vi "H.Signal.vi"() -> (2 "element":bool, 4 "Slide servo home RS":bool, 6 "HI Bit Auto":bool, 8 "Error M Auto":string, 10 "Error Message":string, 15 "Bool_H Sig":bool)   [LabVIEW 2015]
uses:
  Galobal variable_TI.vi
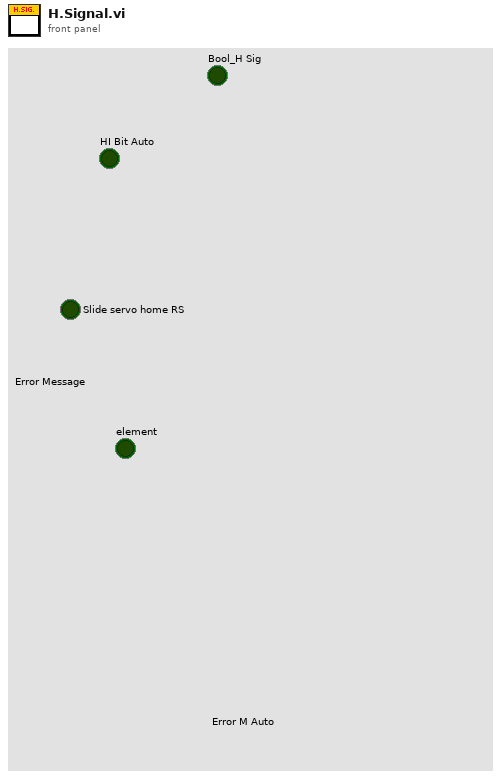
[diagram p1: front panel]
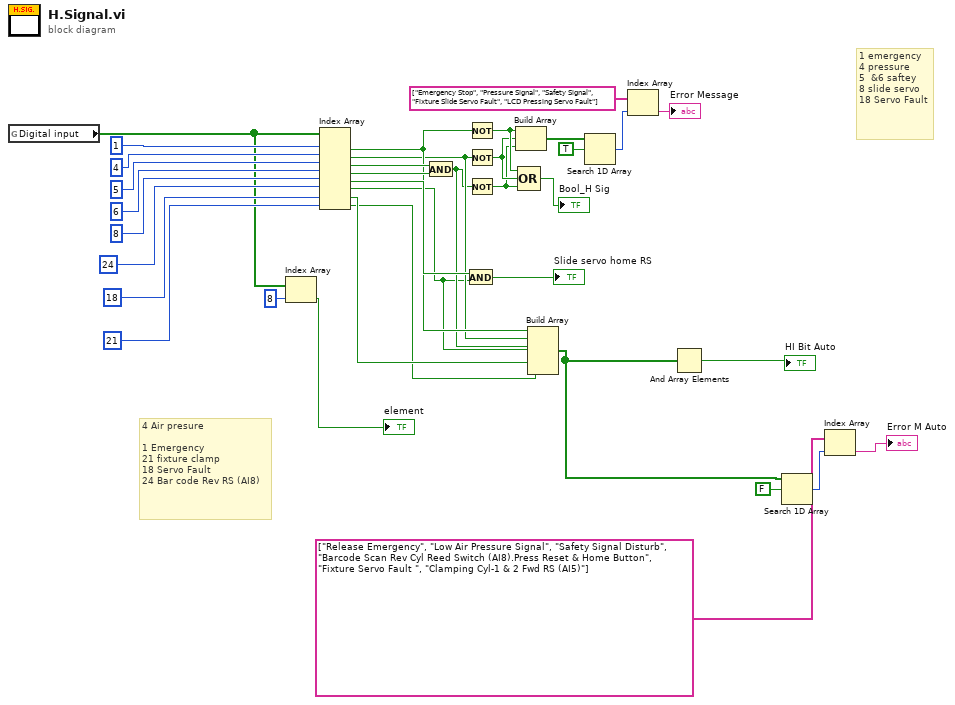
[diagram p0: block diagram]
diagram:
  # "4 Air presure\n  \n1 Emergency\n21 fixture clamp\n18 Servo Fault\n24 Bar code Rev RS (AI8)"
  # "1 emergency\n4 pressure\n5  &6 saftey\n8 slide servo\n18 Servo Fault"
  n1 = global read "Galobal variable_TI.vi" "Digital input"() -> (w3:bool[])
  n2 = Index Array(array=w3, index=8) -> (element=→"element":bool)
  n3 = Index Array(array=w3, index #1=1 ("index"), index #2=4 ("index"), index #3=5 ("index"), index #4=6 ("index"), index #5=8 ("index"), index #6=24 ("index"), index #7=18 ("index"), index #8=21 ("index")) -> (element #1=w17:bool, element #2=w16:bool, element #3=w31:bool, element #4=w30:bool, element #5=w19:bool, element #6=w14:bool, element #7=w8:bool, element #8=w4:bool)
  n4 = And(x=w31, y=w30) -> (x .and. y?=w15:bool)
  n5 = And(x=w19, y=w14) -> (x .and. y?=→"Slide servo home RS":bool)
  n6 = Not(x=w17) -> (.not. x?=w23:bool)
  n7 = Not(x=w16) -> (.not. x?=w22:bool)
  n8 = Not(x=w15) -> (.not. x?=w21:bool)
  n9 = Build Array(w23, w22, w21) -> (w26:bool[])
  n10 = Compound Arithmetic op=OR(w23, w22, w21) -> (→"Bool_H Sig":bool)
  n11 = Build Array(w17, w16, w15, w14, w8, w4) -> (w7:bool[])
  n12 = Search 1D Array(1D array=w26, element=TRUE) -> (index of element=w28:i32)  [unwired: 1 in]
  n13 = Index Array(array=string[] ["Emergency Stop", "Pressure Signal", "Safety Signal", "Fixture Slide Servo Fault", "LCD Pressing Servo Fault"], index=w28) -> (element=→"Error Message":string)
  n14 = And Array Elements(Boolean array=w7) -> (logical AND=→"HI Bit Auto":bool)
  n15 = Search 1D Array(1D array=w7, element=FALSE) -> (index of element=w12:i32)  [unwired: 1 in]
  n16 = Index Array(array=string[] ["Release Emergency", "Low Air Pressure Signal", "Safety Signal Disturb", "Barcode Scan Rev Cyl Reed Switch (AI8).Press Reset & Home Button", "Fixture Servo Fault ", "Clamping Cyl-1 & 2 Fwd RS (AI5)"], index=w12) -> (element=→"Error M Auto":string)
